vi "Test Call Assertion Type Recorded on Passing Pass If Equal.vi"(8 "error in (no error)":errorcluster, 11 "Test Case In":refnum<class "Test Case Assertions Test.lvclass">) -> (0 "error out":errorcluster, 3 "Test Case Out":refnum<class "Test Case Assertions Test.lvclass">)   [LabVIEW 2020, in "Test Case Assertions Test.lvclass"]
uses:
  Test Case Assertions Test.lvclass
  C:/Program Files (x86)/National Instruments/LabVIEW 2020/vi.lib/Astemes/LUnit/Test Case.lvclass
  Test Doubles/Test Case Test Double/Methods.ctl
  source/Core/Result/Type.ctl
  <vilib>/Astemes/LUnit/Test Case.lvclass/Test Case.ctl
  e8c5eeff-a694-4c0d-b261-74e2e6f5327d.vi
  <vilib>/Astemes/LUnit/Append Pass Result.vi
  <vilib>/Astemes/LUnit/Append Fail Result.vi
  <vilib>/Astemes/LUnit/Compare Variants.vi
  <vilib>/Astemes/LUnit/Describe Comparison.vi
  <vilib>/Astemes/LUnit/Variant to string.vi
  <vilib>/Utility/Data Type/Get Type Information.vi
  <vilib>/Utility/LVClass/Get LV Class Name.vi
  source/API/LUnit Test Case/LUnit Test Case.lvclass
  Test Doubles/Test Case Test Double/Test Case Test Double.lvclass
  source/Core/Result/Result.lvlib
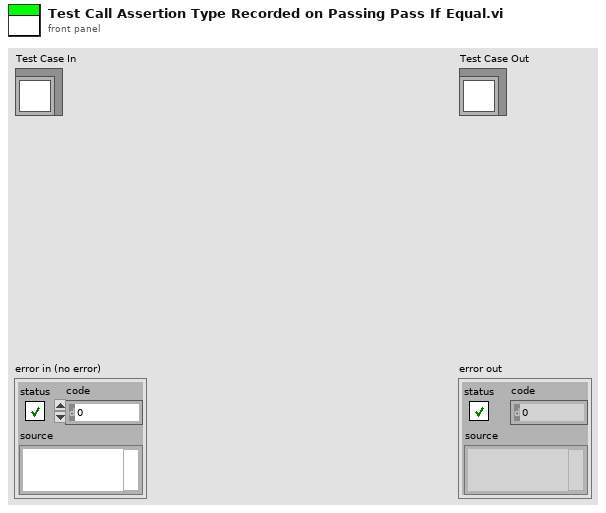
[diagram p1: front panel]
types:
  T1 = typedef "Result.lvlib/Type.ctl" = enum16{"Test Case", "Test Suite", "Test Run", "Pass", "Fail", "Skip", "Pass if", "Fail if", "Pass if Error", "Fail if Error", "Pass if Equal", "Fail if Equal"}
  T2 = typedef "Test Case Test Double.lvclass/Methods.ctl" = enum16{"Test Failing Test.vi", "Test Passing Test.vi", "Test Error Test.vi", "Test Skip Test.vi", "Test Passing Pass If Test.vi", "Test Failing Pass If Test.vi", "Test Failing Fail If Test.vi", "Test Passing Fail If Test.vi", "Test Passing Pass If Error Test.vi", "Test Failing Pass If Error Test.vi", "Test Passing Fail If Error Test.vi", "Test Failing Fail If Error Test.vi", "Test Passing Pass If Equal Test.vi", "Test Failing Pass If Equal Test.vi", "Test Failing Fail If Equal Test.vi", "Test Passing Fail If Equal Test.vi", "Freezing Test.vi"}
  T3 = typedef "Result.lvlib/Result.ctl" = cluster{"Name":string, "Message":string, "Description":string, "Status":T4, "Result Type":T1, "Execution Time":dbl}
  T4 = typedef "Result.lvlib/Status.ctl" = enum16{"", "Passed", "Failed", "Error", "Skipped", "Setup Error", "Broken", "Teardown Error"}
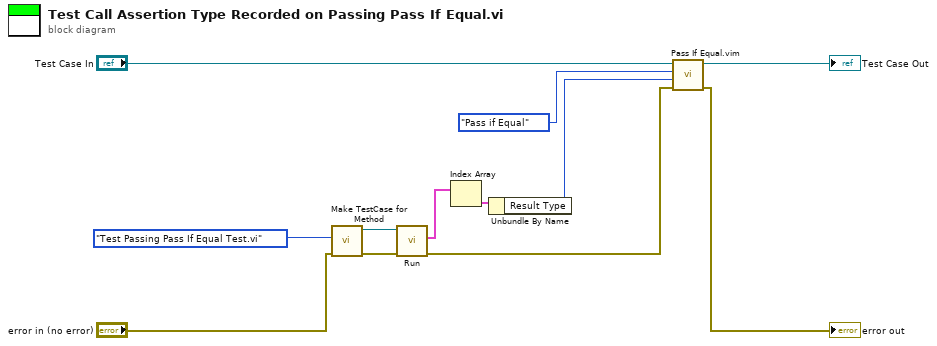
[diagram p0: block diagram]
diagram:
  n1 = call "Make TestCase for Method.vi"("error in (no error)"="error in (no error)", "Test Method"=Methods."Test Passing Pass If Equal Test.vi") -> ("error out"=w8:errorcluster, "LUnit Test Case V2 out"=w9:refnum<class "LUnit Test Case.lvclass">)  [unwired: 8 in]
  n2 = call-dynamic "Run.vi"("error in (no error)"=w8, "LUnit Test Case In"=w9) -> ("error out"=w6:errorcluster, "Results"=w5:T3[])  [unwired: 6 in, 2 out]
  n3 = Index Array(array=w5) -> (element=w4:T3)  [unwired: 1 in]
  n4 = Unbundle By Name(w4) -> ("Result Type"=w3:T1)
  n5 = call "Pass If Equal.vim"("error in (no error)"=w6, "Actual"=w3, "Expected"=Type."Pass if Equal" ("Result Type"), "LUnit Test Case In"="Test Case In") -> ("error out"=→"error out":errorcluster, "LUnit Test Case Out"=→"Test Case Out":refnum<class "Test Case Assertions Test.lvclass">)  [unwired: 6 in]
